vi "Main.vi"() -> (0 "error out":errorcluster, 1 "Aborted":bool)   [LabVIEW 2019]
uses:
  LVMQTT-master/Controls/Connection_Return_Codes.ctl
  LVMQTT-master/Controls/QoS.ctl
  LVMQTT-master/Controls/Retain_Flag.ctl
  LVMQTT-master/Controls/DUP_Flag.ctl
  LVMQTT-master/Controls/Connect_Flags.ctl
  <vilib>/FPGAPlugInAG/sbRIO-9642/niLvFpga_Open_sbRIO-9642.vi
  <vilib>/rvi/interface/common/dynamic/niFpgaDynamicAddResources.vi
  <vilib>/Utility/error.llb/Error Cluster From Error Code.vi
  <vilib>/rvi/errors/niLvFpgaAdjustHostInterfaceError.vi
  <vilib>/rvi/interface/nirviOpenFPGA/nirviOpenFPGA.xnode
  FPGA Bitfiles/sbrio-9642sauna_FPGATarget2_Sauna9642FPGAMai_36EMwFdAsqY.lvbitx
  <vilib>/rvi/interface/nirviReadWriteControl/nirviReadWriteControl.xnode
  LVMQTT-master/MQTT_Functions.lvlib
  <vilib>/NI_Real-Time Target Support.lvlib
  NiFpgaLv.dll
  <vilib>/rvi/interface/Simulation/niFpgaSimulationCallBeginRW.vi
panel:
  out "Vol0":dbl
  out "MessageID":i32
  out "Connection Status":T1=enum."Connection refused: not authorized"
  in  "Stop Publishing":bool
  out "Message":string
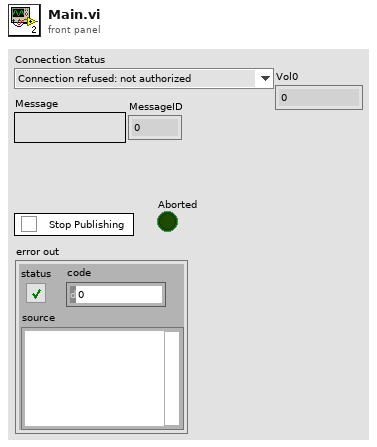
[diagram p1: front panel]
types:
  T1 = typedef "MQTT_Functions.lvlib/Connection_Return_Codes.ctl" = enum16{"Connection accepted", "Connection refused: unacceptable protocol version", "Connection refused: identifier rejected", "Connection refused: Server unavailable", "Connection refused: bad user name or password", "Connection refused: not authorized"}
  T2 = typedef "MQTT_Functions.lvlib/QoS.ctl" = enum8{"At most once", "At least once", "Exactly once", "Reserved"}
  T3 = typedef "MQTT_Functions.lvlib/DUP_Flag.ctl" = bool
  T4 = typedef "MQTT_Functions.lvlib/Retain_Flag.ctl" = bool
  T5 = cluster{"QoS":T2, "DUP":T3, "Retain":T4, "Keep Alive (sec)":u16}
  T6 = typedef "MQTT_Functions.lvlib/Connect_Flags.ctl" = cluster{"user name":bool, "password":bool, "will retain":bool, "will flag":bool, "clean session":bool, "reserved":bool, "will QoS":T2}
  T7 = cluster{"Temp0":dbl, "Temp1":dbl, "Temp2":dbl, "Vol0":dbl, "Sw0":bool}
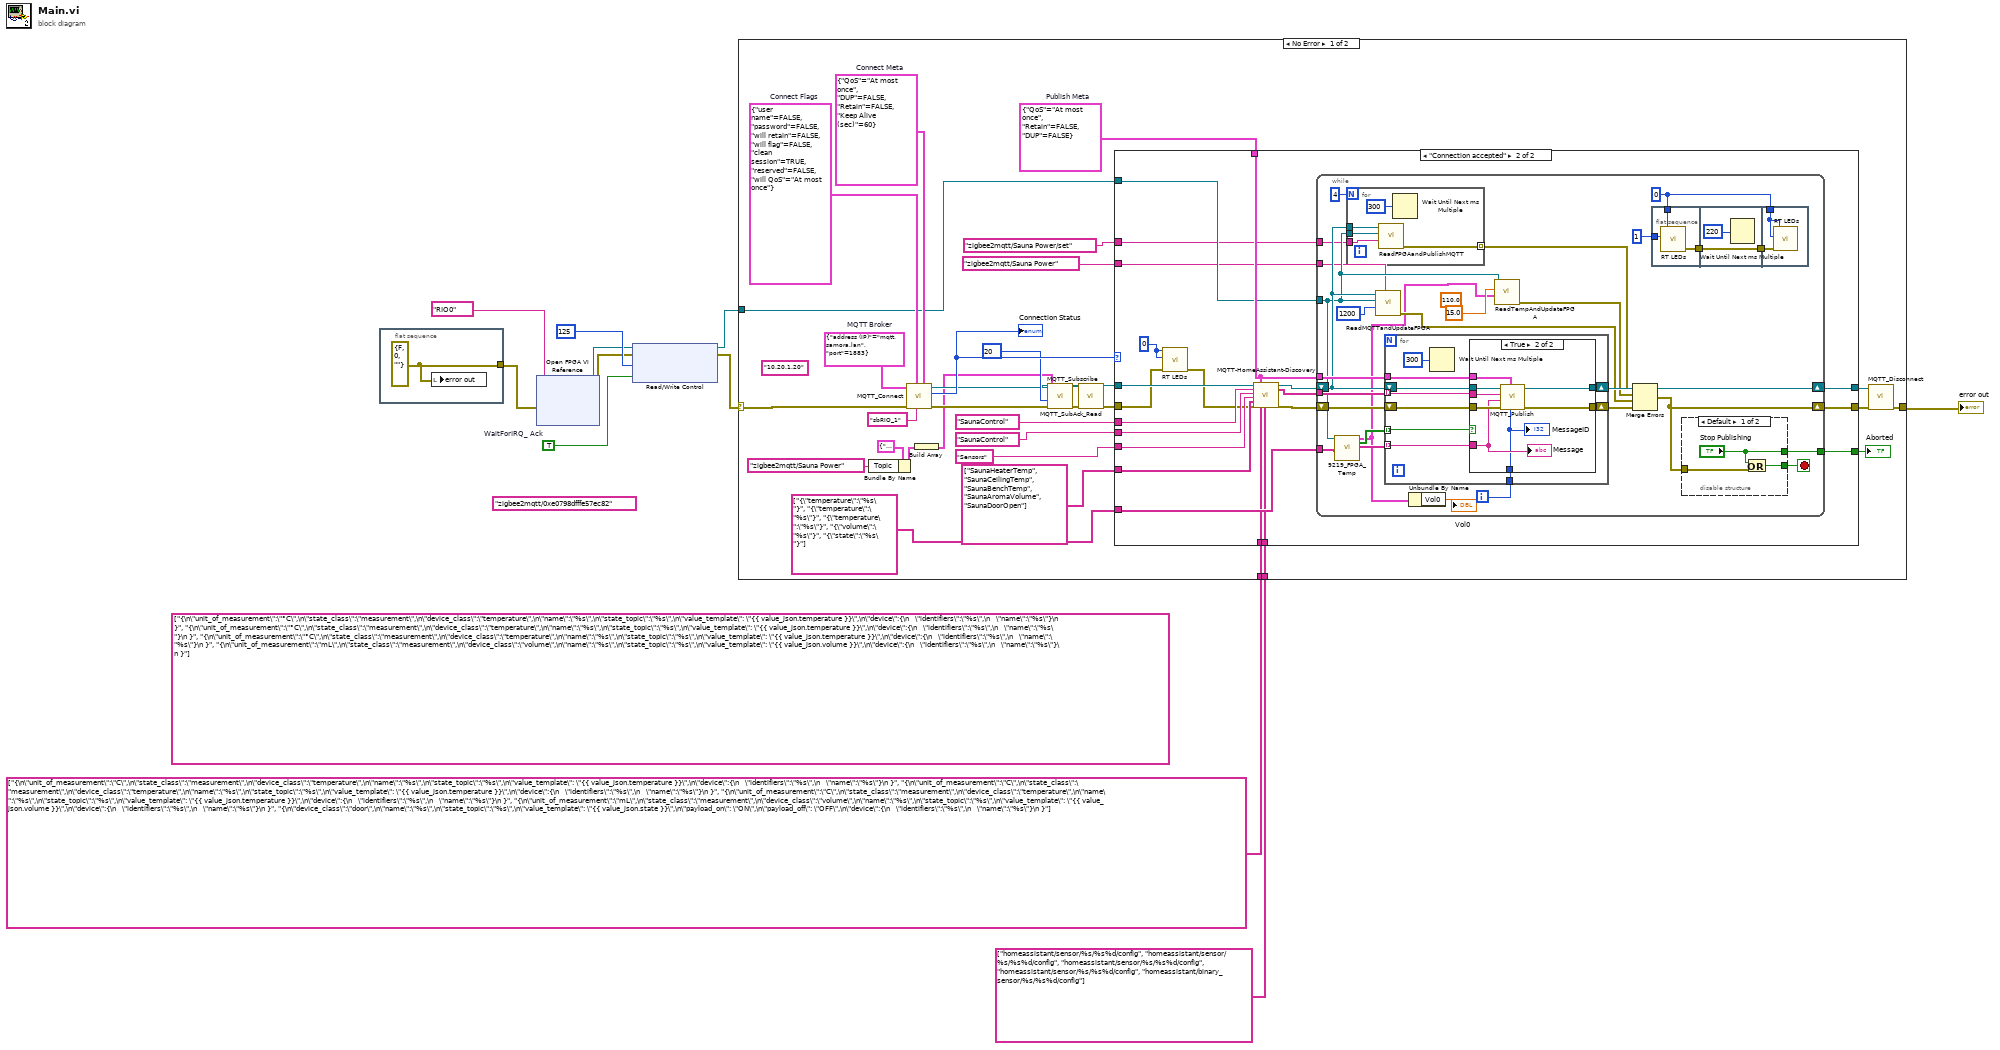
[diagram p0: block diagram]
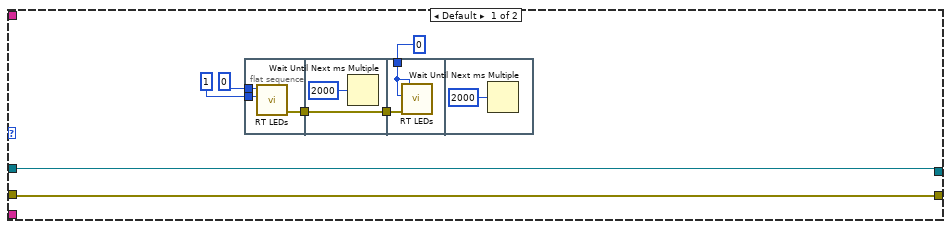
[diagram p2: hidden frame]
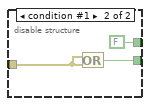
[diagram p3: hidden frame]
diagram:
  (unwired) "zigbee2mqtt/0xe0798dfffe57ec82" ("Topic")
  (unwired) string[] ["{\n\"unit_of_measurement\":\"°C\",\n\"state_class\":\"measurement\",\n\"device_class\":\"temperature\",\n\"name\":\"%s\",\n\"state_topic\":\"%s\",\n\"value_template\": \"{{ value_json.temperature }}\",\n\"device\":{\n   \"identifiers\":\"%s\",\n   \"name\":\"%s\"}\n }", "{\n\"unit_of_measurement\":\"°C\",\n\"state_class\":\"measurement\",\n\"device_class\":\"temperature\",\n\"name\":\"%s\",\n\"state_topic\":\"%s\",\n\"value_template\": \"{{ value_json.temperature }}\",\n\"device\":{\n   \"identifiers\":\"%s\",\n   \"name\":\"%s\"}\n }", "{\n\"unit_of_measurement\":\"°C\",\n\"state_class\":\"measurement\",\n\"device_class\":\"temperature\",\n\"name\":\"%s\",\n\"state_topic\":\"%s\",\n\"value_template\": \"{{ value_json.temperature }}\",\n\"device\":{\n   \"identifiers\":\"%s\",\n   \"name\":\"%s\"}\n }", "{\n\"unit_of_measurement\":\"mL\",\n\"state_class\":\"measurement\",\n\"device_class\":\"volume\",\n\"name\":\"%s\",\n\"state_topic\":\"%s\",\n\"value_template\": \"{{ value_json.volume }}\",\n\"device\":{\n   \"identifiers\":\"%s\",\n   \"name\":\"%s\"}\n }"]
  w3 = TRUE  # WaitForIRQ_ Ack
  n1 = flat-sequence {
    tunnel: [w12] -> w9
    frame #0 {
      w12 = errorcluster {"status"=FALSE, "code"=0, "source"=""} ("error in (no error)")
      n2 = local write "error out"(w12) -> ()
    }
  }
  n3 = xnode "Open FPGA VI Reference"("error in"=w9, "resource name"=tag "RIO0") -> ("FPGA VI Reference Out"=w7:refnum<k20>, "error out"=w5:errorcluster)
  n4 = xnode "Read/Write Control"("FPGA VI Reference In"=w7, "error in"=w5, "Pump Cycle"=u32 125, "WaitForIRQ_ Ack"=w3) -> ("FPGA VI Reference Out"=w6:refnum<k20>, "error out"=w4:errorcluster)
  n5 = case shown="No Error" w4 {
    selector: w4 -> [w22 w147]
    tunnel: [w41 w147] -> w11
    tunnel: w6 -> [w23 _]
    tunnel: string[] ["{\n\"unit_of_measurement\":\"C\",\n\"state_class\":\"measurement\",\n\"device_class\":\"temperature\",\n\"name\":\"%s\",\n\"state_topic\":\"%s\",\n\"value_template\": \"{{ value_json.temperature }}\",\n\"device\":{\n   \"identifiers\":\"%s\",\n   \"name\":\"%s\"}\n }", "{\n\"unit_of_measurement\":\"C\",\n\"state_class\":\"measurement\",\n\"device_class\":\"temperature\",\n\"name\":\"%s\",\n\"state_topic\":\"%s\",\n\"value_template\": \"{{ value_json.temperature }}\",\n\"device\":{\n   \"identifiers\":\"%s\",\n   \"name\":\"%s\"}\n }", "{\n\"unit_of_measurement\":\"C\",\n\"state_class\":\"measurement\",\n\"device_class\":\"temperature\",\n\"name\":\"%s\",\n\"state_topic\":\"%s\",\n\"value_template\": \"{{ value_json.temperature }}\",\n\"device\":{\n   \"identifiers\":\"%s\",\n   \"name\":\"%s\"}\n }", "{\n\"unit_of_measurement\":\"mL\",\n\"state_class\":\"measurement\",\n\"device_class\":\"volume\",\n\"name\":\"%s\",\n\"state_topic\":\"%s\",\n\"value_template\": \"{{ value_json.volume }}\",\n\"device\":{\n   \"identifiers\":\"%s\",\n   \"name\":\"%s\"}\n }", "{\n\"device_class\":\"door\",\n\"name\":\"%s\",\n\"state_topic\":\"%s\",\n\"value_template\": \"{{ value_json.state }}\",\n\"payload_on\": \"ON\",\n\"payload_off\": \"OFF\",\n\"device\":{\n   \"identifiers\":\"%s\",\n   \"name\":\"%s\"}\n }"] -> [w20 _]
    tunnel: string[] ["homeassistant/sensor/%s/%s%d/config", "homeassistant/sensor/%s/%s%d/config", "homeassistant/sensor/%s/%s%d/config", "homeassistant/sensor/%s/%s%d/config", "homeassistant/binary_sensor/%s/%s%d/config"] -> [w13 _]
    frame No Error {
      (unwired) "10.20.1.20" ("address (IP)")
      w42 = T5 {"QoS"=enum."At most once", "DUP"=FALSE, "Retain"=FALSE, "Keep Alive (sec)"=60}  # Connect Meta
      w44 = T6 {"user name"=FALSE, "password"=FALSE, "will retain"=FALSE, "will flag"=FALSE, "clean session"=TRUE, "reserved"=FALSE, "will QoS"=enum."At most once"}  # Connect Flags
      w37 = cluster{"address (IP)":string, "port":u16} {"address (IP)"="mqtt.samora.lan", "port"=1883}  # MQTT Broker
      w40 = cluster{"QoS":T2, "Retain":T4, "DUP":T3} {"QoS"=enum."At most once", "Retain"=FALSE, "DUP"=FALSE}  # Publish Meta
      n6 = Bundle By Name(cluster=cluster{"Topic":string, "QoS":T2} {"Topic"="zigbee2mqtt/0xe0798dfffe57ec82", "QoS"=enum."At most once"} ("Subscription Info"), "Topic"="zigbee2mqtt/Sauna Power") -> (w17:cluster{"Topic":string, "QoS":T2})
      n7 = call "MQTT_Connect.vi"("Connect Meta"=w42, "Client ID"="sbRIO_1", "Connect Flags"=w44, "error in (no error)"=w22, "MQTT Broker"=w37) -> ("error out"=w25:errorcluster, "Connection Status"=w36:T1, "connection ID out"=w27:refnum<k5>)  [unwired: 4 in]
      "Connection Status" <- w36
      n8 = Build Array(w17) -> (w18:cluster{"Topic":string, "QoS":T2}[])
      n9 = call "MQTT_Subscribe.vi"("error in (no error)"=w25, "Message ID"=u16 20, "Subscription Info Array"=w18, "connection ID"=w27) -> ("error out"=w28:errorcluster, "connection ID out"=w29:refnum<k5>)  [unwired: 6 in]
      n10 = call "MQTT_SubAck_Read.vi"("error in (no error)"=w28, "connection ID"=w29) -> ("error out"=w24:errorcluster, "connection ID out"=w26:refnum<k5>)  [unwired: 7 in, 1 out]
      n11 = case shown="\"Connection accepted\"" w36 {
        tunnel: w40 -> [_ w73]
        tunnel: [w50 w80] -> w39
        tunnel: [w51 w79] -> w38
        tunnel: w24 -> [w50 w67]
        tunnel: w26 -> [w51 w78]
        tunnel: string[] ["{\"temperature\":\"%s\"}", "{\"temperature\":\"%s\"}", "{\"temperature\":\"%s\"}", "{\"volume\":\"%s\"}", "{\"state\":\"%s\"}"] ("ChannelNames") -> [_ w74]
        tunnel: string[] ["SaunaHeaterTemp", "SaunaCeilingTemp", "SaunaBenchTemp", "SaunaAromaVolume", "SaunaDoorOpen"] ("ChannelNames") -> [_ w69]
        tunnel: "SaunaControl" ("Device") -> [_ w72]
        tunnel: "SaunaControl" ("DeviceName") -> [_ w71]
        tunnel: "Sensors" ("ChannelBase") -> [_ w70]
        tunnel: [_ w65] -> w31
        tunnel: w23 -> [_ w64]
        tunnel: w20 -> [_ w63]
        tunnel: "zigbee2mqtt/Sauna Power/set" ("Topic") -> [_ w62]
        tunnel: "zigbee2mqtt/Sauna Power" ("Topic") -> [_ w61]
        tunnel: w13 -> [_ w60]
        frame Default {
          n12 = flat-sequence {
            tunnel: [w54] -> w49
            tunnel: 1 ("State") -> [w53]
            tunnel: 0 ("State") -> [w52]
            tunnel: w49 -> [w56]
            tunnel: [w56] -> w48
            tunnel: w48 -> [w58]
            tunnel: 0 ("State") -> [w57]
            frame #0 {
              n13 = call <vilib>:"RT LEDs.vi"("State"=w53, "LED Num"=w52) -> ("error out"=w54:errorcluster)  [unwired: 4 in, 1 out]
            }
            frame #1 {
              n14 = Wait Until Next ms Multiple(millisecond multiple=u32 2000) -> ()  [unwired: 1 out]
            }
            frame #2 {
              n15 = call <vilib>:"RT LEDs.vi"("error in (no error)"=w58, "State"=w57, "LED Num"=w57) -> ()  [unwired: 3 in, 2 out]
            }
            frame #3 {
              n16 = Wait Until Next ms Multiple(millisecond multiple=u32 2000) -> ()  [unwired: 1 out]
            }
          }
        }
        frame "Connection accepted" {
          w66 = 0 ("State")
          n17 = call <vilib>:"RT LEDs.vi"("error in (no error)"=w67, "State"=w66, "LED Num"=w66) -> ("error out"=w68:errorcluster)  [unwired: 3 in, 1 out]
          n18 = call "MQTT-HomeAssistant-Discovery.vi"("TCP Network Connection in"=w78, "Device"=w72, "DeviceName"=w71, "ChannelBase"=w70, "ChannelNames"=w69, "error in (no error)"=w68, "Publish Meta"=w73, "MessageTemplate"=w63, "ConfigPath"=w60) -> ("TCP Network Connection out"=w76:refnum<k5>, "Topics"=w75:string[], "error out"=w77:errorcluster)  [unwired: 8 in]
          n19 = while {
            tunnel: w73 -> [w107]
            shift-right: [w96] -> w80
            shift-left: w77 -> [w108]
            shift-right: [w106] -> w79
            shift-left: w76 -> [w92]
            tunnel: w75 -> [w102]
            tunnel: w74 -> [w88]
            tunnel: [w98] -> w65
            tunnel: w64 -> [w85]
            tunnel: w62 -> [w82]
            tunnel: w61 -> [w81]
            i -> [w103]
            stop <- w105 stop-if-true
            (unwired) 110.0 ("TempThreshold")
            w97 = 0 ("State")
            n20 = call "9219_FPGA_Temp.vi"("FPGA VI Reference"=w85, "MessageFormats"=w88) -> ("Sensors"=w83:T7, "updated?"=w86:bool[], "Messages"=w87:string[])  [unwired: 14 in, 1 out]
            n21 = for {
              N: 4 -> [_]
              tunnel: w92 -> [w112]
              tunnel: w85 -> [w111]
              tunnel: [w110] -> w91 mode=indexing
              tunnel: w82 -> [w109]
              n22 = call "ReadFPGAandPublishMQTT.vi"("Topic"=w109, "FPGA VI Reference"=w111, "MQTT"=w112) -> ("error out"=w110:errorcluster)  [unwired: 7 in, 1 out]
              n23 = Wait Until Next ms Multiple(millisecond multiple=u32 300) -> ()  [unwired: 1 out]
            }
            n24 = call "ReadMQTTandUpdateFPGA.vi"("Topic"=w81, "timeout ms (25000)"=1200, "FPGA VI Reference"=w85, "MQTT"=w92) -> ("error out"=w95:errorcluster)  [unwired: 7 in]
            n25 = for {
              tunnel: w107 -> [w134]
              tunnel: w86 -> [w131] mode=indexing
              shift-right: [w133] -> w106
              shift-left: w92 -> [w136]
              shift-right: [w132] -> w104
              shift-left: w108 -> [w135]
              tunnel: w87 -> [w130] mode=indexing
              tunnel: w103 -> [w128]
              tunnel: w102 -> [w127] mode=indexing
              n26 = Wait Until Next ms Multiple(millisecond multiple=u32 300) -> ()  [unwired: 1 out]
              n27 = case shown="True" w131 {
                tunnel: w127 -> [_ w146]
                tunnel: w136 -> [w138 w145]
                tunnel: w135 -> [w137 w144]
                tunnel: w134 -> [_ w143]
                tunnel: [w138 w142] -> w133
                tunnel: [w137 w141] -> w132
                tunnel: w130 -> [_ w140]
                tunnel: w128 -> [_ w139]
                frame False {
                }
                frame True {
                  n28 = call "MQTT_Publish.vi"("Message ID"=w139, "Publish Meta"=w143, "error in (no error)"=w144, "Message to be published"=w140, "Topic"=w146, "connection ID"=w145) -> ("error out"=w141:errorcluster, "connection ID out"=w142:refnum<k5>)  [unwired: 4 in]
                  "Message" <- w140
                  "MessageID" <- w139
                }
              }
            }
            n29 = Unbundle By Name(w83) -> ("Vol0"=→"Vol0":dbl)
            n30 = call "ReadTempAndUpdateFPGA.vi"("Sensors"=w83, "TempThreshold"=15.0, "FPGA VI Reference"=w85) -> ("error out"=w90:errorcluster)  [unwired: 8 in]
            n31 = Merge Errors(w91, w90, w95, w104) -> (w96:errorcluster)
            n32 = flat-sequence {
              tunnel: [w116] -> w101
              tunnel: 1 ("State") -> [w115]
              tunnel: w97 -> [w114]
              tunnel: w101 -> [w118]
              tunnel: [w118] -> w100
              tunnel: w100 -> [w120]
              tunnel: w97 -> [w119]
              frame #0 {
                n33 = call <vilib>:"RT LEDs.vi"("State"=w115, "LED Num"=w114) -> ("error out"=w116:errorcluster)  [unwired: 4 in, 1 out]
              }
              frame #1 {
                n34 = Wait Until Next ms Multiple(millisecond multiple=u32 220) -> ()  [unwired: 1 out]
              }
              frame #2 {
                n35 = call <vilib>:"RT LEDs.vi"("error in (no error)"=w120, "State"=w119, "LED Num"=w119) -> ()  [unwired: 3 in, 2 out]
              }
            }
            n36 = disable-structure shown="Default" {
              disable-tunnel: [w123 w126] -> w105
              disable-tunnel: w96 -> [w122 w125]
              disable-tunnel: ["Stop Publishing" FALSE ("Stop Publishing")] -> w98
              frame condition #0 (active) {
                n37 = Or(x="Stop Publishing", y=w122) -> (x .or. y?=w123:bool)
              }
              frame condition #1 {
                n38 = Or(x=w125, y=w125) -> (x .or. y?=w126:bool)
              }
            }
          }
        }
      }
      "Aborted" <- w31
      n39 = call "MQTT_Disconnect.vi"("error in (no error)"=w39, "connection ID"=w38) -> ("error out"=w41:errorcluster)  [unwired: 9 in]
    }
    frame Error {
    }
  }
  "error out" <- w11
